vi "initArray.vi"(10 "dim":i32, 11 "element":dbl) -> (3 "Array":dbl[](array[numeric]))   [LabVIEW 2020]
panel:
  out "error out":errorcluster
  in  "error in (no error)":errorcluster
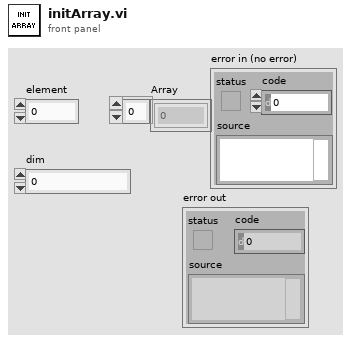
[diagram p1: front panel]
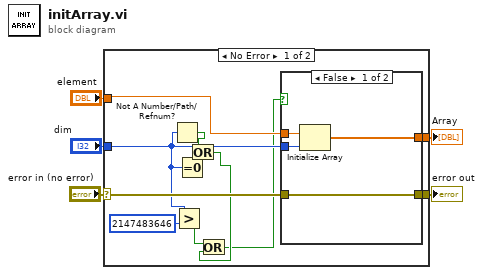
[diagram p0: block diagram]
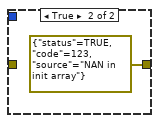
[diagram p2: hidden frame]
diagram:
  n1 = case shown="No Error" "error in (no error)" {
    selector: "error in (no error)" -> [w14 w22]
    tunnel: "dim" -> [w10 _]
    tunnel: "element" -> [w16 _]
    tunnel: [w15 _] -> w3
    tunnel: [w13 w22] -> w1
    frame No Error {
      n2 = Not A Number/Path/Refnum?(number/path/refnum=w10) -> (NaN/Path/Refnum?=w12:bool)
      n3 = Greater?(x=w10, y=2147483646) -> (0:w8:bool)
      n4 = Equal To 0?(x=w10) -> (x = 0?=w11:bool)
      n5 = Or(x=w12, y=w11) -> (x .or. y?=w7:bool)
      n6 = Or(x=w8, y=w7) -> (x .or. y?=w6:bool)
      n7 = case shown="False" w6 {
        tunnel: w16 -> [w20 _]
        tunnel: w10 -> [w19 _]
        tunnel: [w18 _] -> w15
        tunnel: w14 -> [w17 _]
        tunnel: [w17 errorcluster {"status"=TRUE, "code"=123, "source"="NAN in init array"} ("error IO")] -> w13
        frame False {
          n8 = Initialize Array(w20, w19) -> (w18:dbl[])
        }
        frame True {
        }
      }
    }
    frame Error {
    }
  }
  "error out" <- w1
  "Array" <- w3
